vi "Host.vi"   [LabVIEW 2025]
uses:
  <vilib>/Handler Framework/CmdQueue/Enqueue Single.vi
  <vilib>/Handler Framework/Handler Framework.lvlib
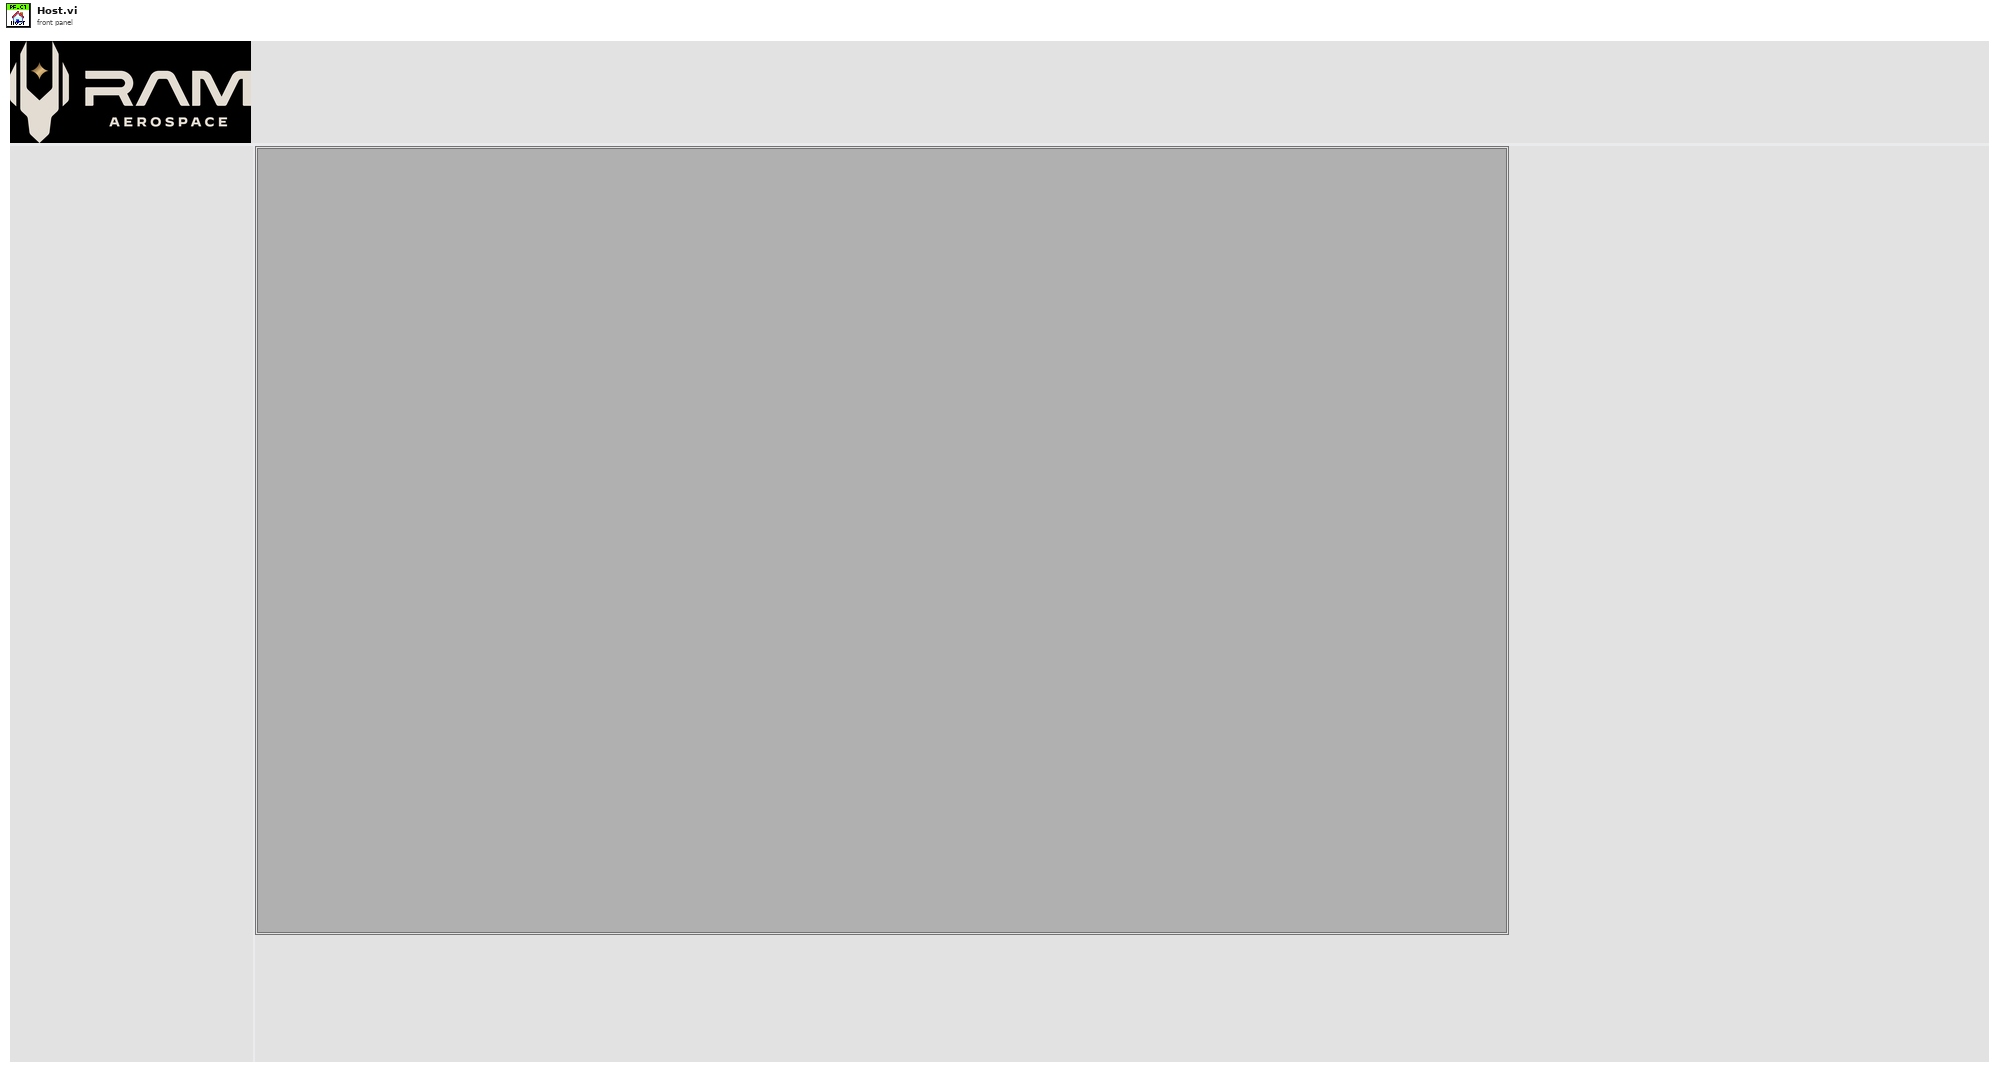
[diagram p1: front panel]
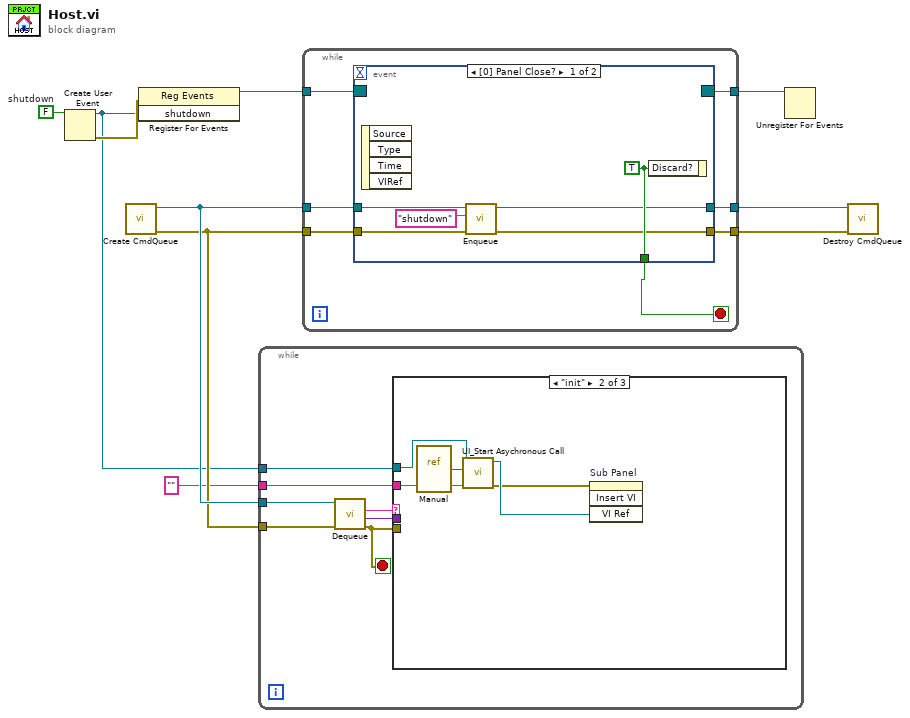
[diagram p0: block diagram]
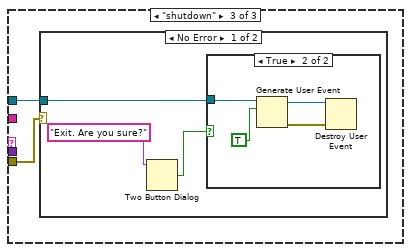
[diagram p3: hidden frame]
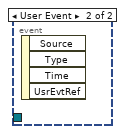
[diagram p6: hidden frame]
diagram:
  w6 = FALSE  # shutdown
  n1 = Create User Event(user event datatype=w6) -> (user event=w1:refnum<user-event>, error out=w2:errorcluster)  [unwired: 1 in]
  n2 = call <vilib>:"Create CmdQueue.vi"() -> ("error out"=w7:errorcluster, "CmdQueue out"=w8:refnum<queue>)  [unwired: 10 in]
  n3 = register-events(error in=w2, w1) -> (reference out=w5:refnum<event-registration>)  [unwired: 1 in, 1 out]
  n4 = while {
    tunnel: w8 -> [w17]
    tunnel: w7 -> [w14]
    tunnel: w1 -> [w13]
    tunnel: "" ("String") -> [w12]
    stop <- w11 stop-if-true
    n5 = call <vilib>:"Dequeue.vi"("error in (no error)"=w14, "CmdQueue in"=w17) -> ("error out"=w11:errorcluster, "value"=w15:variant, "cmd"=w16:string)  [unwired: 5 in, 2 out]
    n6 = case shown="\"init\"" w16 {
      tunnel: w15 -> [_ _ _]
      tunnel: w13 -> [_ w19 w24]
      tunnel: w12 -> [_ w18 _]
      tunnel: w11 -> [_ _ w23]
      frame "False", Default {
      }
      frame "init" {
        n7 = vi-ref "Manual.vi"() -> (w22:refnum<vi>)
        n8 = call "UI_Start Asychronous Call.vi"("String"=w18, "VI Refnum"=w22, "User Event in"=w19) -> ("error out"=w20:errorcluster, "VI out"=w21:refnum<vi>)  [unwired: 7 in]
        n9 = invoke on="Sub Panel" class="SubPnl" method="Insert VI"(error in=w20, "VI Ref"=w21) -> ()  [unwired: 2 in, 4 out]
      }
      frame "shutdown" {
        n10 = case shown="No Error" w23 {
          tunnel: w24 -> [w25 _]
          frame No Error {
            n11 = Two Button Dialog(message="Exit. Are you sure?") -> (T button?=w26:bool)  [unwired: 2 in]
            n12 = case shown="True" w26 {
              tunnel: w25 -> [_ w31]
              frame False {
              }
              frame True {
                n13 = Generate User Event(user event=w31, event data cluster=TRUE ("event data")) -> (user event out=w29:refnum<user-event>, error out=w28:errorcluster)  [unwired: 2 in]
                n14 = Destroy User Event(user event=w29, error in=w28) -> ()  [unwired: 1 out]
              }
            }
          }
          frame Error {
          }
        }
      }
    }
  }
  n15 = while {
    tunnel: w8 -> [w36]
    tunnel: [w34] -> w10
    tunnel: w7 -> [w35]
    tunnel: [w33] -> w9
    tunnel: w5 -> [w38]
    tunnel: [w37] -> w4
    stop <- w32 stop-if-true
    n16 = event shown="[0] Panel Close?" {
      selector: w38 -> [_ _]
      dyn-events: [_ _] -> w37
      timeout: _ -> [_ _]
      tunnel: w36 -> [w43 _]
      tunnel: w35 -> [w42 _]
      tunnel: [w40 _] -> w34
      tunnel: [w39 _] -> w33
      tunnel: [w41 _] -> w32
      event Panel Close? {
        w41 = TRUE ("Discard?")
        n17 = event-data() -> ()  [unwired: 1 in, 4 out]
        n18 = call-poly <vilib>:"Enqueue.vi"("error in (no error)"=w42, "Command"="shutdown", "CmdQueue in"=w43) -> ("error out"=w39:errorcluster, "CmdQueue out"=w40:refnum<queue>)  [unwired: 7 in]
        n19 = event-data("Discard?"=w41) -> ()  [unwired: 1 in, 1 out]
      }
      event User Event {
        n20 = event-data() -> ()  [unwired: 1 in, 4 out]
      }
    }
  }
  n21 = Unregister For Events(event registration refnum=w4) -> ()  [unwired: 1 in, 1 out]
  n22 = call <vilib>:"Destroy CmdQueue.vi"("error in (no error)"=w9, "CmdQueue in"=w10) -> ()  [unwired: 9 in, 1 out]
